vi "Get Circles.vi"(8 "error in (no error)":errorcluster, 11 "ParseSVG in":refnum<class "ParseSVG.lvclass">) -> (0 "error out":errorcluster, 3 "ParseSVG out":refnum<class "ParseSVG.lvclass">)   [LabVIEW 2019, in "ParseSVG.lvclass"]
uses:
  ParseSVG.lvclass
  Dot.ctl
  ParseSVG.lvclass/ParseSVG.ctl
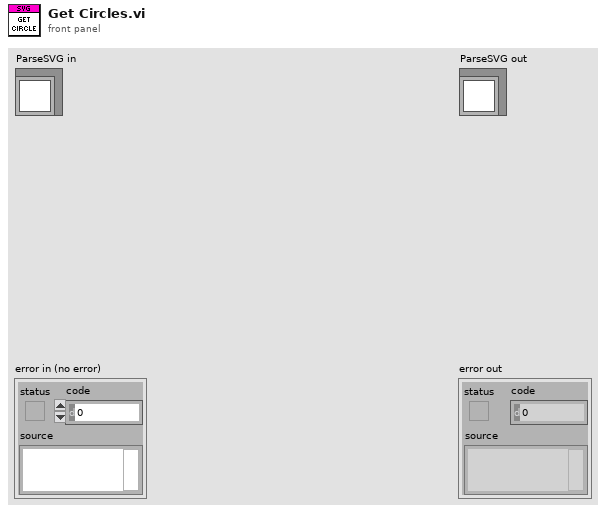
[diagram p1: front panel]
types:
  T1 = typedef "ParseSVG.lvclass/Dot.ctl" = cluster{"cx":string, "cy":string, "r":string, "style":string, "id":string}
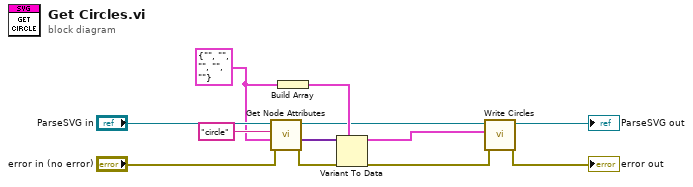
[diagram p0: block diagram]
diagram:
  w1 = T1 {"cx"="", "cy"="", "r"="", "style"="", "id"=""} ("circle")
  n1 = call "Get Node Attributes.vi"("error in (no error)"="error in (no error)", "Attributes Cluster"=w1, "Node Name (exact)"="circle", "ParseSVG in"="ParseSVG in") -> ("error out"=w7:errorcluster, "[Attributes Cluster]"=w9:variant[], "ParseSVG out"=w6:refnum<class "ParseSVG.lvclass">)  [unwired: 5 in]
  n2 = Build Array(w1) -> (w8:T1[])
  n3 = Variant To Data(error in=w7, type=w8, Variant=w9) -> (data=w2:T1[], error out=w4:errorcluster)
  n4 = call "Write Circles.vi"("error in (no error)"=w4, "Circles"=w2, "ParseSVG in"=w6) -> ("error out"=→"error out":errorcluster, "ParseSVG out"=→"ParseSVG out":refnum<class "ParseSVG.lvclass">)  [unwired: 7 in]
